vi "CThread Get Completed CRef.vi"(4 "index":i32) -> (1 "CRef: Complete?":T1)   [LabVIEW 2012, in "CThread.lvlib"]
uses:
  CThread.lvlib
  CRef/Interface/CRef Boolean.llb/Boolean CReference.ctl
  CRef/CRef.lvlib
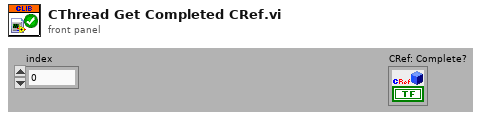
[diagram p1: front panel]
types:
  T1 = typedef "CRef.lvlib/Boolean CReference.ctl" = cluster{"Boolean CRef Address":u16, "Type":enum8{"Null", "Boolean", "U8", "I8", "U16", "I16", "U32", "I32", "U64", "I64", "Single", "Double", "Extended", "CSG", "CDB", "CXT", "Boolean(Def)"}}
  T2 = typedef "CThread.lvlib/CThread Governor Data.ctl" = cluster{"Action":enum16{"Inactive", "While Loop", "For Loop", "Do When Loop", "Scheduled"}, "End Delay":u32, "Requested Runs":u32, "Completion Index":u16, "Conditional Index":u16}
  T3 = typedef "CRef.lvlib/Variant CReference.ctl" = cluster{"Generic CRef Address":u16, "Type":u8}
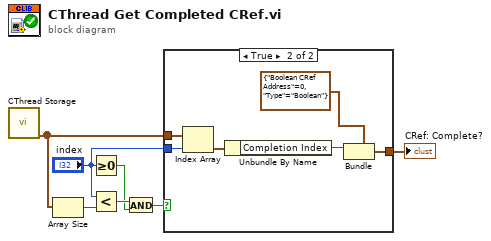
[diagram p0: block diagram]
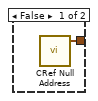
[diagram p2: hidden frame]
diagram:
  n1 = call "CThread Storage.vi"() -> ("Governer Table"=w5:T2[])  [unwired: 10 in, 5 out]
  n2 = Array Size(array=w5) -> (size(s)=w6:i32)
  n3 = Greater Or Equal To 0?(x="index") -> (x >= 0?=w2:bool)
  n4 = Less?(x="index", y=w6) -> (x < y?=w3:bool)
  n5 = And(x=w3, y=w2) -> (x .and. y?=w1:bool)
  n6 = case shown="True" w1 {
    tunnel: w5 -> [_ w14]
    tunnel: "index" -> [_ w13]
    tunnel: [w8 w11] -> w7
    frame False {
      n7 = call "CRef Null Address.vi"() -> ("Null CReference"=w8:T3)  [unwired: 5 in]
    }
    frame True {
      n8 = Index Array(array=w14, index=w13) -> (element=w10:T2)
      n9 = Unbundle By Name(w10) -> ("Completion Index"=w9:u16)
      n10 = Bundle(cluster=T1 {"Boolean CRef Address"=0, "Type"=enum."Boolean"} ("Boolean CReference"), "Boolean CRef Address"=w9) -> (w11:T1)  [unwired: 1 in]
    }
  }
  "CRef: Complete?" <- w7
